vi "CSM - Add VI Reference Case to CSMs.vi"() -> ()   [LabVIEW 2017]
doc: "The CSM template must include the \"VI Reference\" branch for external access to VI references. In early templates, this case was not included, and this tool is used to add it.\n\nThis tool scans all VIs in the lvproj directory; if a VI contains a CSM module, it will be listed, and then you can choose to batch add the \"VI Reference\" branch."
uses:
  user.lib/_NEVSTOP/Communicable State Machine(CSM)/AdvanceAPI/CSM - Make String Arguments Safe.vi
  user.lib/_NEVSTOP/Communicable State Machine(CSM)/_Support/Common/Format Timestamp.vi
  user.lib/_NEVSTOP/Communicable State Machine(CSM)/AdvanceAPI/CSM - Keywords.vi
  user.lib/_NEVSTOP/Communicable State Machine(CSM)/Communicable State Machine.lvlib
  user.lib/_NEVSTOP/Communicable State Machine(CSM)/_csmHelper/Utility/CSM-Helper Utility.lvlib
  user.lib/_NEVSTOP/Communicable State Machine(CSM)/_tool/_ui/csm-ui-support.lvlib
panel:
  out "Serarching Path":path
  in  "Stop Searching":bool
  in  "add":bool
  in  "Show FP?":bool=TRUE
  out "Array":path[](array[path])
  out "String":string
  out "Slide":i32(slide) scale=0.0..100.0
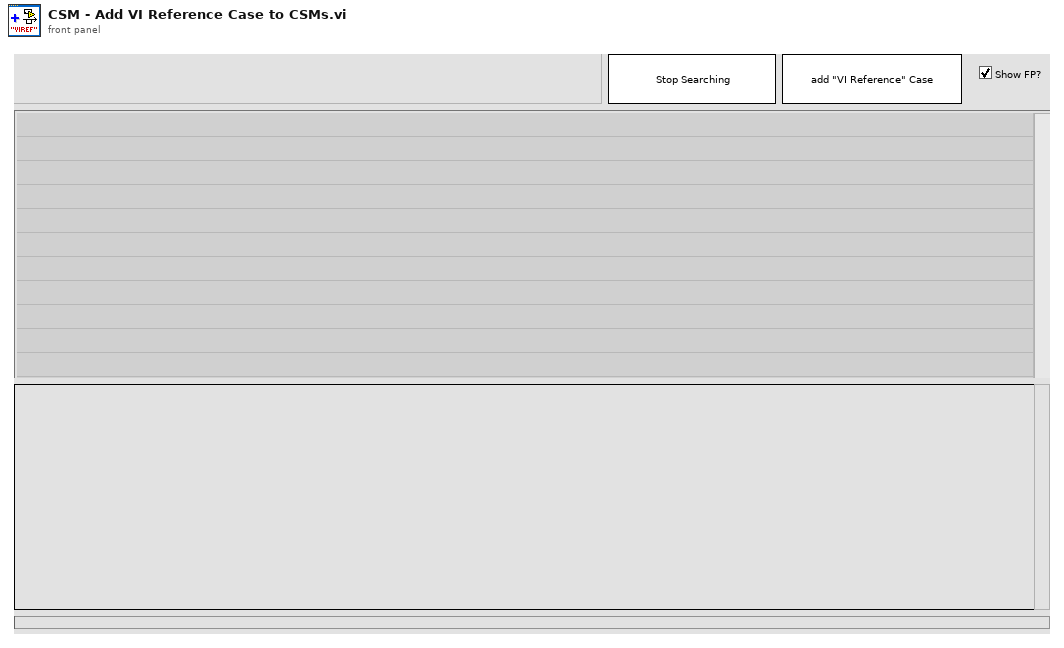
[diagram p1: front panel]
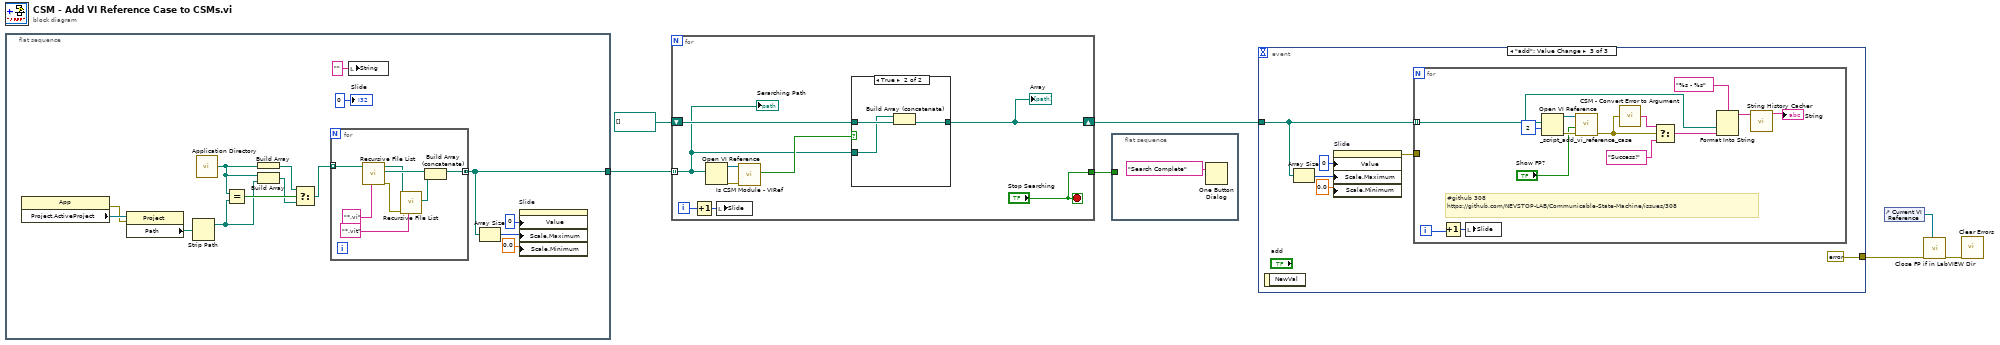
[diagram p0: block diagram]
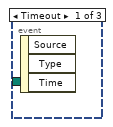
[diagram p3: hidden frame]
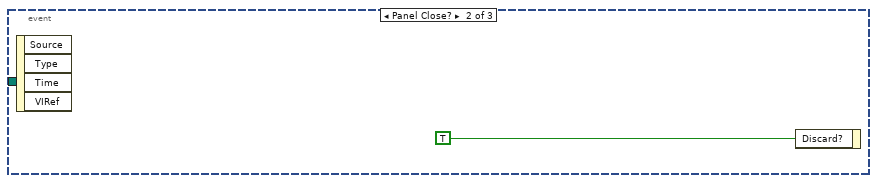
[diagram p4: hidden frame]
diagram:
  n1 = flat-sequence {
    tunnel: [w8] -> w4
    frame #0 {
      n2 = property class="App"() -> (error out=w21:errorcluster, "Project.ActiveProject"=w22:refnum<vi>)  [unwired: 2 in, 1 out]
      n3 = property class="Project"(reference=w22, error in=w21) -> ("Path"=w20:path)  [unwired: 2 out]
      n4 = Strip Path(path=w20) -> (stripped path=w16:path)  [unwired: 1 out]
      n5 = call <vilib>:"Application Directory.vi"() -> ("Application Directory"=w17:path)
      n6 = Equal?(x=w17, y=w16) -> (x = y?=w19:bool)
      n7 = Build Array(w17) -> (w18:path[])
      n8 = Build Array(w17, w16) -> (w15:path[])
      n9 = Select(t=w18, s=w19, f=w15) -> (s? t:f=w14:path[])
      n10 = for {
        tunnel: [w25] -> w8 mode=concatenating
        tunnel: w14 -> [w23] mode=indexing
        n11 = call <vilib>:"Recursive File List.vi"("pattern"="*.vi", "Folder Path"=w23) -> ("error out"=w27:errorcluster, "All Files in Dir"=w29:path[], "dup Folder Path"=w26:path)  [unwired: 5 in, 2 out]
        n12 = call <vilib>:"Recursive File List.vi"("pattern"="*.vit", "error in (no error)"=w27, "Folder Path"=w26) -> ("All Files in Dir"=w24:path[])  [unwired: 4 in, 4 out]
        n13 = Build Array (concatenate)(w29, w24) -> (w25:path[])
      }
      n14 = local write "String"("" ("String")) -> ()
      n15 = Array Size(array=w8) -> (size(s)=w9:i32)
      n16 = property on="Slide" class="Slide (strict)"("Value"=0 ("Slide"), "Scale.Maximum"=w9, "Scale.Minimum"=0.0 ("Scale.Range:Minimum")) -> ()  [unwired: 2 in, 2 out]
      "Slide" <- 0 ("Slide")
    }
  }
  n17 = for {
    tunnel: w4 -> [w34] mode=indexing
    shift-right: [w33] -> w6
    shift-left: path[] [] -> [w39]
    tunnel: ["Stop Searching"] -> w5
    i -> [w32]
    stop <- "Stop Searching" stop-if-true
    n18 = Increment(x=w32) -> (x+1=w31:i32)
    n19 = Open VI Reference(vi path=w34) -> (vi reference=w38:refnum<vi>, error out=w37:errorcluster)  [unwired: 5 in]
    n20 = local write "Slide"(w31) -> ()
    n21 = call "Is CSM Module - VIRef.vi"("error in (no error)"=w37, "VIRef"=w38) -> ("Is CSM Module?"=w35:bool)  [unwired: 6 in, 3 out]
    n22 = case shown="True" w35 {
      tunnel: w39 -> [w40 w43]
      tunnel: w34 -> [_ w42]
      tunnel: [w40 w41] -> w33
      frame False {
      }
      frame True {
        n23 = Build Array (concatenate)(w42, w43) -> (w41:path[])
      }
    }
    "Array" <- w33
    "Serarching Path" <- w34
  }
  n24 = flat-sequence {
    tunnel: w5 -> [_]
    frame #0 {
      n25 = One Button Dialog(message="Search Complete") -> ()  [unwired: 1 in, 1 out]
    }
  }
  n26 = event shown="[2] \"add\": Value Change" {
    selector: _ -> [_ _ _]
    dyn-events: _ -> [_ _ _]
    timeout: _ -> [_ _ _]
    tunnel: w6 -> [_ _ w48]
    tunnel: [_ _ errorcluster {"status"=FALSE, "code"=0, "source"=""} ("Error in")] -> w1
    event Timeout {
      n27 = event-data() -> ()  [unwired: 1 in, 3 out]
    }
    event Panel Close? {
      n28 = event-data() -> ()  [unwired: 1 in, 4 out]
      n29 = event-data("Discard?"=TRUE) -> ()  [unwired: 1 in, 1 out]
    }
    event "add": Value Change {
      n30 = event-data() -> ()  [unwired: 1 in, 1 out]
      n31 = Array Size(array=w48) -> (size(s)=w51:i32)
      n32 = property on="Slide" class="Slide (strict)"("Value"=0 ("Slide"), "Scale.Maximum"=w51, "Scale.Minimum"=0.0 ("Scale.Range:Minimum")) -> (error out=w47:errorcluster)  [unwired: 2 in, 1 out]
      n33 = for {
        tunnel: w48 -> [w59] mode=indexing
        tunnel: w47 -> [_]
        i -> [w52]
        # "#github 308 \nhttps://github.com/NEVSTOP-LAB/Communicable-State-Machine/issues/308"
        n34 = Increment(x=w52) -> (x+1=w53:i32)
        n35 = local write "Slide"(w53) -> ()
        n36 = Open VI Reference(vi path=w59, options=2) -> (vi reference=w65:refnum<vi>, error out=w64:errorcluster)  [unwired: 4 in]
        n37 = call "_script_add_vi_reference_case.vi"("error in (no error)"=w64, "Show FP?"="Show FP?", "VI Ref"=w65) -> ("error out"=w63:errorcluster)  [unwired: 8 in]
        n38 = call "CSM - Convert Error to Argument.vi"("Error"=w63) -> ("Argument"=w62:string)  [unwired: 4 in]
        n39 = Select(t=w62, s=w63, f="Success!") -> (s? t:f=w60:string)
        n40 = Format Into String(format string="%s - %s", w59, w60) -> (resulting string=w57:string)  [unwired: 2 in, 1 out]
        n41 = call "String History Cacher.vi"("String"=w57) -> ("String Cache"=→"String":string)  [unwired: 10 in]
      }
    }
  }
  n42 = control-ref of="Current VI Reference"() -> (w2:refnum<vi>)
  n43 = call "Close FP if in LabVIEW Dir.vi"("VI Refnum"=w2, "Error in"=w1) -> ("Error out"=w3:errorcluster)  [unwired: 9 in]
  n44 = call <vilib>:"Clear Errors.vi"("error in (no error)"=w3) -> ()  [unwired: 5 in, 2 out]
